vi "CreateMessageBus.vi"() -> (3 "MessageQueues":T1)   [LabVIEW 2024]
uses:
  MessageQueues.ctl
  <vilib>/httpClient/ClientHandle.ctl
  <vilib>/httpClient/LabVIEWHTTPClient.lvlib
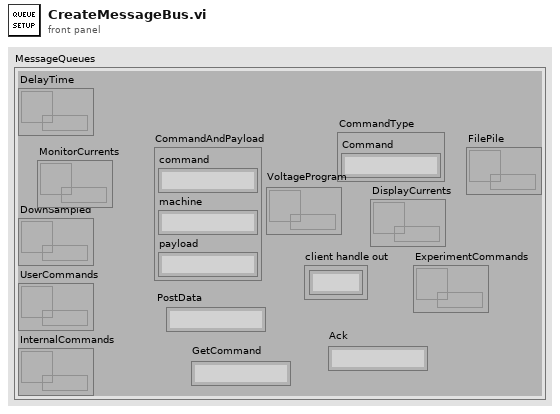
[diagram p1: front panel]
types:
  T1 = typedef "MessageQueues.ctl" = cluster{"DelayTime":refnum<queue>, "DownSampled":refnum<queue>, "UserCommands":refnum<queue>, "InternalCommands":refnum<queue>, "CommandType":cluster{"Command":string}, "CommandAndPayload":cluster{"command":string, "machine":string, "payload":string}, "client handle out":T2, "PostData":string, "GetCommand":string, "Ack":string, "VoltageProgram":refnum<queue>, "ExperimentCommands":refnum<queue>, "DisplayCurrents":refnum<queue>, "MonitorCurrents":refnum<queue>, "FilePile":refnum<queue>}
  T2 = typedef "LabVIEWHTTPClient.lvlib/ClientHandle.ctl" = refnum<k1>
  T3 = cluster{"Waveforms":waveform(dbl)[], "file":refnum<k34>}
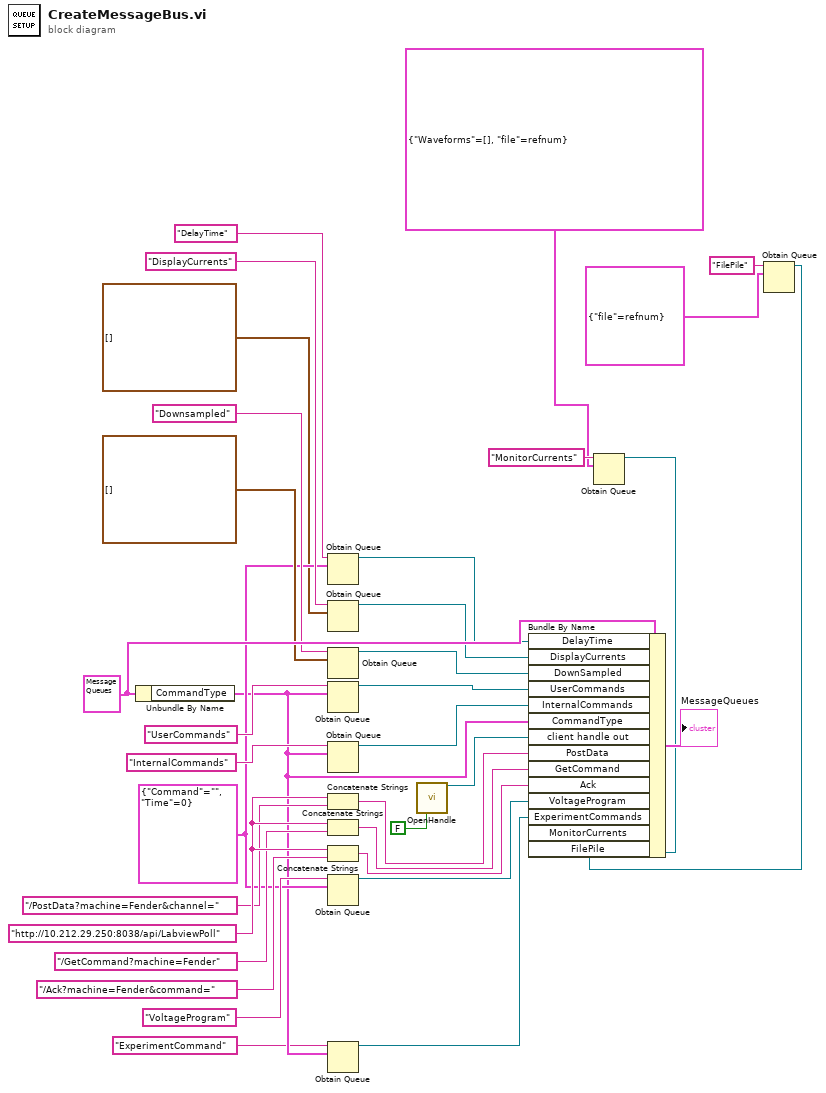
[diagram p0: block diagram]
diagram:
  w31 = T1 {"DelayTime"=refnum, "DownSampled"=refnum, "UserCommands"=refnum, "InternalCommands"=refnum, "CommandType"={"Command"=""}, "CommandAndPayload"={"command"="", "machine"="", "payload"=""}, "client handle out"=refnum, "PostData"="", "GetCommand"="", "Ack"="", "VoltageProgram"=refnum, "ExperimentCommands"=refnum, "DisplayCurrents"=refnum, "MonitorCurrents"=refnum, "FilePile"=refnum}
  w23 = "http://10.212.29.250:8038/api/LabviewPoll"
  w12 = cluster{"Command":string, "Time":i32} {"Command"="", "Time"=0}
  n1 = Unbundle By Name(w31) -> ("CommandType"=w10:cluster{"Command":string})
  n2 = Obtain Queue(name (unnamed)="DelayTime", element data type=w12) -> (queue out=w25:refnum<queue>)  [unwired: 3 in, 2 out]
  n3 = Obtain Queue(name (unnamed)="DisplayCurrents", element data type=waveform(dbl)[] []) -> (queue out=w26:refnum<queue>)  [unwired: 3 in, 2 out]
  n4 = Obtain Queue(name (unnamed)="Downsampled", element data type=waveform(dbl)[] []) -> (queue out=w29:refnum<queue>)  [unwired: 3 in, 2 out]
  n5 = Obtain Queue(name (unnamed)="UserCommands", element data type=w10) -> (queue out=w28:refnum<queue>)  [unwired: 3 in, 2 out]
  n6 = Obtain Queue(name (unnamed)="InternalCommands", element data type=w10) -> (queue out=w27:refnum<queue>)  [unwired: 3 in, 2 out]
  n7 = Concatenate Strings(w23, "/PostData?machine=Fender&channel=" ("url")) -> (w33:string)
  n8 = Concatenate Strings(w23, "/GetCommand?machine=Fender" ("url")) -> (w34:string)
  n9 = Concatenate Strings(w23, "/Ack?machine=Fender&command=" ("url")) -> (w35:string)
  n10 = Obtain Queue(name (unnamed)="VoltageProgram", element data type=w12) -> (queue out=w11:refnum<queue>)  [unwired: 3 in, 2 out]
  n11 = Obtain Queue(name (unnamed)="ExperimentCommand", element data type=w10) -> (queue out=w8:refnum<queue>)  [unwired: 3 in, 2 out]
  n12 = call <vilib>:"OpenHandle.vi"("verify server(true)"=FALSE) -> ("client handle out"=w32:T2)  [unwired: 13 in, 1 out]
  n13 = Obtain Queue(name (unnamed)="MonitorCurrents", element data type=T3 {"Waveforms"=[], "file"=refnum}) -> (queue out=w5:refnum<queue>)  [unwired: 3 in, 2 out]
  n14 = Obtain Queue(name (unnamed)="FilePile", element data type=cluster{"file":refnum<k34>} {"file"=refnum}) -> (queue out=w1:refnum<queue>)  [unwired: 3 in, 2 out]
  n15 = Bundle By Name(cluster=w31, "DelayTime"=w25, "DisplayCurrents"=w26, "DownSampled"=w29, "UserCommands"=w28, "InternalCommands"=w27, "CommandType"=w10, "client handle out"=w32, "PostData"=w33, "GetCommand"=w34, "Ack"=w35, "VoltageProgram"=w11, "ExperimentCommands"=w8, "MonitorCurrents"=w5, "FilePile"=w1) -> (→"MessageQueues":T1)
